vi "Circle.vi"(1 "MaxArray":dbl[][](array[numeric])) -> (0 "Center":cluster{dbl, dbl, dbl})   [LabVIEW 2014]
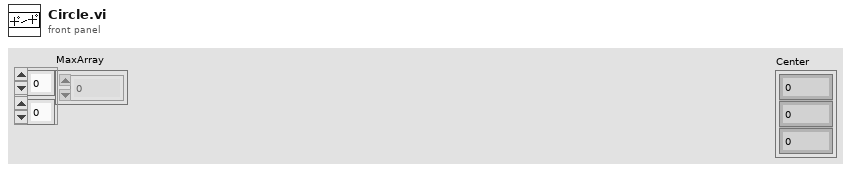
[diagram p1: front panel]
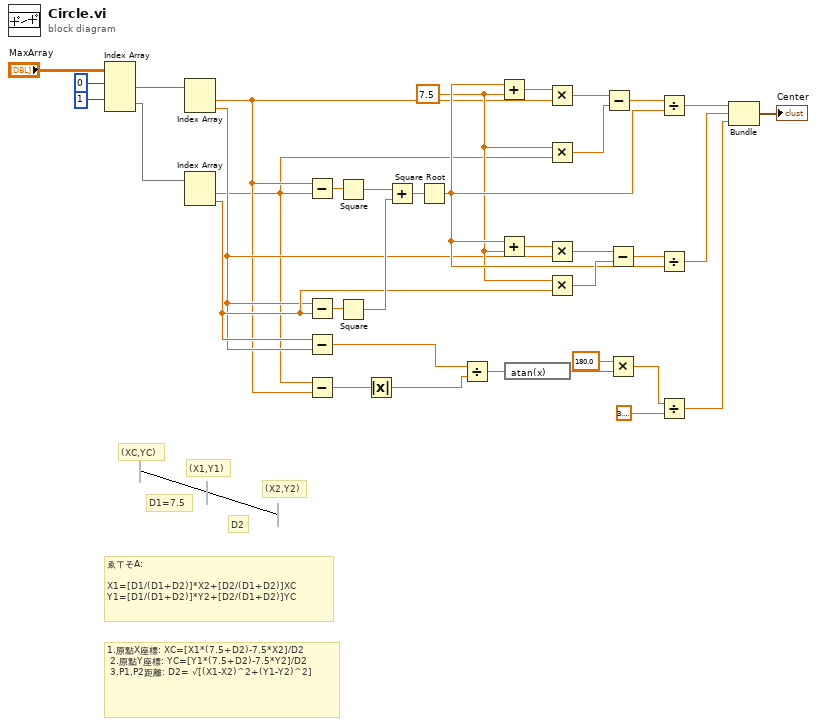
[diagram p0: block diagram]
diagram:
  w17 = 7.5 ("y")
  # "ゑㄒそΑ: \n\nX1=[D1/(D1+D2)]*X2+[D2/(D1+D2)]XC\nY1=[D1/(D1+D2)]*Y2+[D2/(D1+D2)]YC"
  # "D2"
  # "D1=7.5"
  # "(X2,Y2)"
  # "(X1,Y1)"
  # "(XC,YC)"
  # "1.原點X座標: XC=[X1*(7.5+D2)-7.5*X2]/D2     \n 2.原點Y座標: YC=[Y1*(7.5+D2)-7.5*Y2]/D2 \n 3.P1,P2距離: D2= √[(X1-X2)^2+(Y1-Y2)^2]"
  n1 = Index Array(array="MaxArray", index (row) #1=0 ("index (row)"), index (row) #2=1 ("index (row)")) -> (element #1=w19:dbl[], element #2=w18:dbl[])  [unwired: 2 in]
  n2 = Index Array(array=w19) -> (element #1=w10:dbl, element #2=w11:dbl)  [unwired: 2 in]
  n3 = Index Array(array=w18) -> (element #1=w9:dbl, element #2=w12:dbl)  [unwired: 2 in]
  n4 = Subtract(x=w10, y=w9) -> (x-y=w36:dbl)
  n5 = Subtract(x=w11, y=w12) -> (x-y=w35:dbl)
  n6 = Subtract(x=w12, y=w11) -> (x-y=w14:dbl)
  n7 = Subtract(x=w9, y=w10) -> (x-y=w15:dbl)
  n8 = Square(x=w36) -> (x^2=w34:dbl)
  n9 = Square(x=w35) -> (x^2=w33:dbl)
  n10 = Absolute Value(x=w15) -> (abs(x)=w13:dbl)
  n11 = Add(x=w34, y=w33) -> (x+y=w32:dbl)
  n12 = Square Root(x=w32) -> (sqrt(x)=w23:dbl)
  n13 = Divide(x=w14, y=w13) -> (x/y=w8:dbl)
  n14 = Add(x=w23, y=w17) -> (x+y=w31:dbl)
  n15 = Add(x=w23, y=w17) -> (x+y=w24:dbl)
  n16 = expression code="atan(x)"(w8) -> (w7:dbl)
  n17 = Multiply(x=w31, y=w10) -> (x*y=w30:dbl)
  n18 = Multiply(x=w17, y=w9) -> (x*y=w29:dbl)
  n19 = Multiply(x=w24, y=w11) -> (x*y=w25:dbl)
  n20 = Multiply(x=w17, y=w12) -> (x*y=w26:dbl)
  n21 = Subtract(x=w30, y=w29) -> (x-y=w28:dbl)
  n22 = Subtract(x=w25, y=w26) -> (x-y=w27:dbl)
  n23 = Multiply(x=180.0, y=w7) -> (x*y=w5:dbl)
  n24 = Divide(x=w28, y=w23) -> (x/y=w16:dbl)
  n25 = Divide(x=w27, y=w23) -> (x/y=w2:dbl)
  n26 = Divide(x=w5, y=3.141592653589793) -> (x/y=w3:dbl)
  n27 = Bundle(w16, w2, w3) -> (→"Center":cluster{dbl, dbl, dbl})  [unwired: 1 in]
